vi "Set_DO.vi"(8 "error in (no error)":errorcluster, 9 "DO":bool, 10 "PIN":i8, 11 "DI_DO in":refnum<class "DI_DO.lvclass">) -> (0 "error out":errorcluster, 3 "DI_DO out":refnum<class "DI_DO.lvclass">)   [LabVIEW 2023, in "Driver_DI_DO.lvlib" / "DI_DO.lvclass"]
uses:
  DI_DO.lvclass
  DI_DO.lvclass/DI_DO.ctl
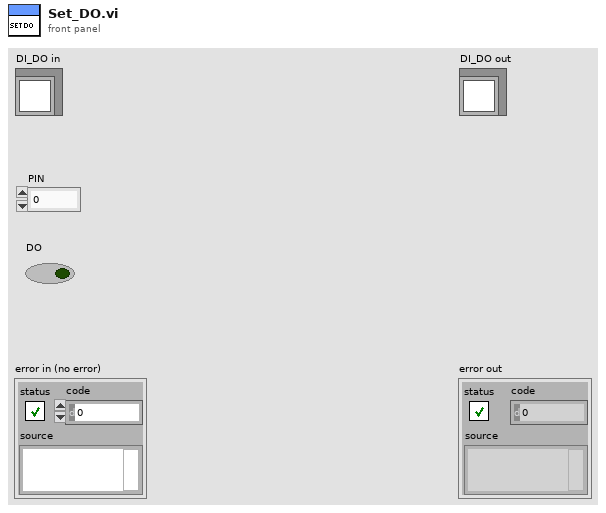
[diagram p1: front panel]
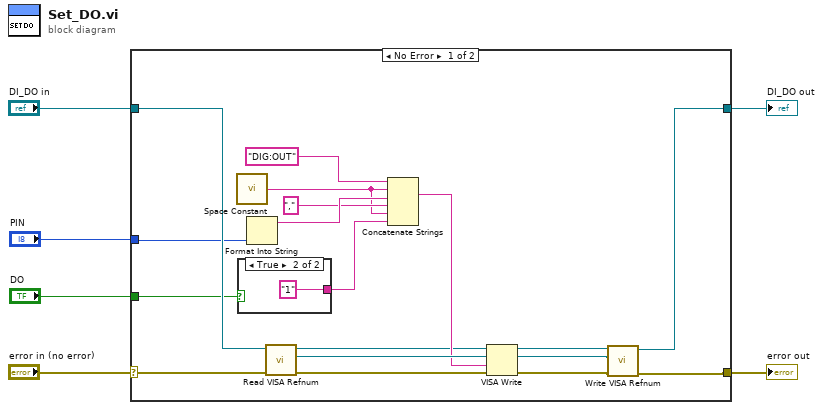
[diagram p0: block diagram]
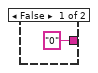
[diagram p2: hidden frame]
diagram:
  n1 = case shown="No Error" "error in (no error)" {
    selector: "error in (no error)" -> [w23 w27]
    tunnel: [w14 w27] -> w5
    tunnel: [w11 w26] -> w3
    tunnel: "DI_DO in" -> [w22 w26]
    tunnel: "DO" -> [w8 _]
    tunnel: "PIN" -> [w19 _]
    frame No Error {
      n2 = call <vilib>:"Space Constant.vi"() -> ("String"=w9:string)
      n3 = case shown="True" w8 {
        tunnel: ["0" "1"] -> w7
        frame False {
        }
        frame True {
        }
      }
      n4 = Format Into String(w19) -> (resulting string=w17:string)  [unwired: 3 in, 1 out]
      n5 = call-dynamic "Read VISA Refnum.vi"("error in (no error)"=w23, "Driver in"=w22) -> ("error out"=w21:errorcluster, "VISA Refnum"=w20:refnum<visa-resource-name>, "Driver out"=w12:refnum<class "DI_DO.lvclass">)  [unwired: 7 in]
      n6 = Concatenate Strings("DIG:OUT" ("string"), w9, w17, ",", w9, w7) -> (w16:string)
      n7 = VISA Write(VISA resource name=w20, write buffer=w16, error in (no error)=w21) -> (VISA resource name out=w13:refnum<visa-resource-name>, error out=w15:errorcluster)  [unwired: 1 out]
      n8 = call-dynamic "Write VISA Refnum.vi"("error in (no error)"=w15, "VISA Refnum"=w13, "Driver in"=w12) -> ("error out"=w14:errorcluster, "Driver out"=w11:refnum<class "DI_DO.lvclass">)  [unwired: 7 in]
    }
    frame Error {
    }
  }
  "error out" <- w5
  "DI_DO out" <- w3
